vi "Handle Messages.vi"(8 "error in (no error)":errorcluster, 9 "Message Data":variant, 10 "Message":string, 11 "Process In":refnum<class "Debugger.lvclass">) -> (0 "error out":errorcluster, 3 "Process Out":refnum<class "Debugger.lvclass">)   [LabVIEW 2020, in "Debugger.lvclass"]
doc: "This is the core VI handling incomming messages to the process. This VI should be overridden to add functionality to the process or override functionality implemented by a parent. Any message not handled should be sent to the parent method using the default case. \nEach state should be atomic and states should in general avoid enqueueing new messages from within this method, as there might be other messages interleaved in the queue from the outside. For cyclic iteration of an action, using a Helper Loop is recommended."
uses:
  Debugger.lvclass
  C:/Git/astemes-triarc-debugger/source/Process/Debug Process.lvclass
  Debug Data/Debug Data.lvclass
  Debugger.lvclass/Debugger.ctl
  Debug Log/Debug Log.lvclass/Debug Log.ctl
  Process/Debug Process.lvclass/Debug Process.ctl
  Process/Public/Lifecycle/Get Lifecycle State.vi
  <vilib>/Utility/error.llb/Clear Errors.vi
  <vilib>/Utility/error.llb/Error Cluster From Error Code.vi
  Process/Debug Process.lvclass
  Debug Log/Debug Log.lvclass
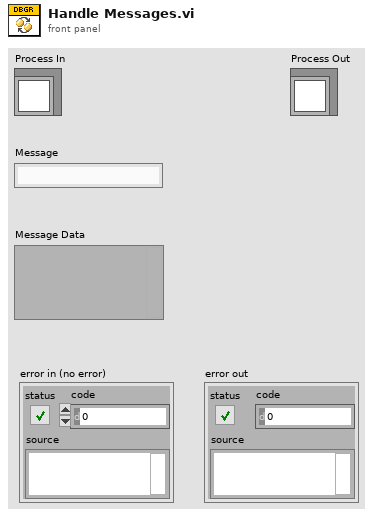
[diagram p1: front panel]
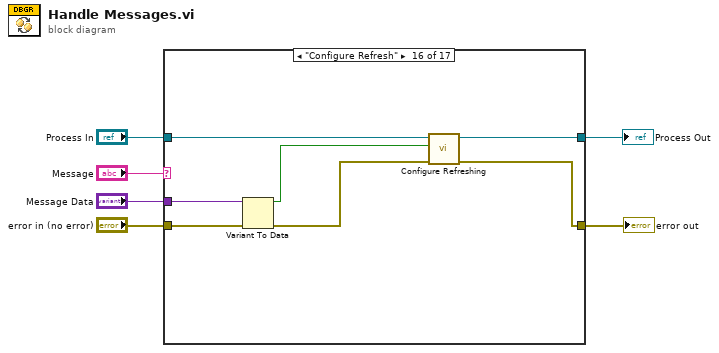
[diagram p0: block diagram]
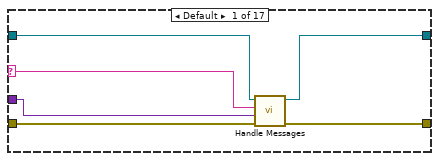
[diagram p2: hidden frame]
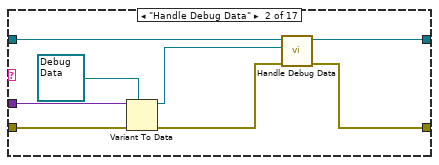
[diagram p3: hidden frame]
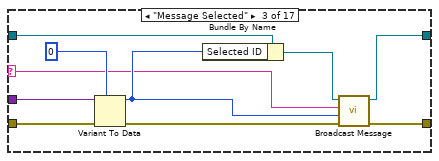
[diagram p4: hidden frame]
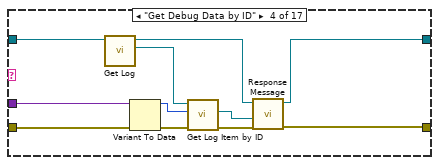
[diagram p5: hidden frame]
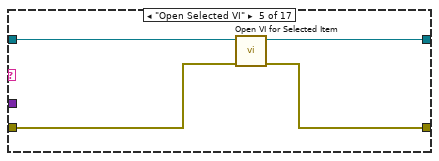
[diagram p6: hidden frame]
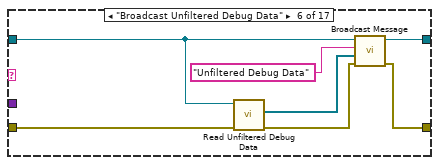
[diagram p7: hidden frame]
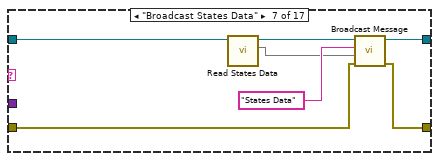
[diagram p8: hidden frame]
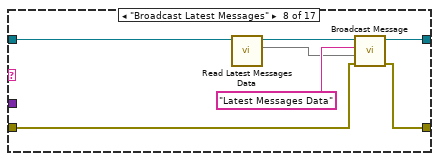
[diagram p9: hidden frame]
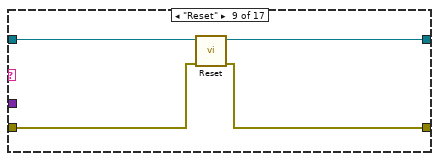
[diagram p10: hidden frame]
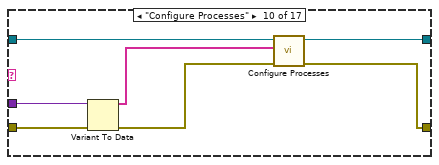
[diagram p11: hidden frame]
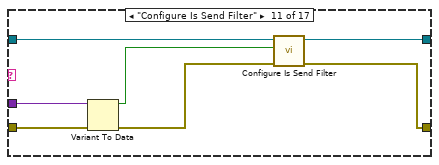
[diagram p12: hidden frame]
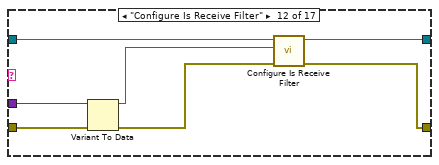
[diagram p13: hidden frame]
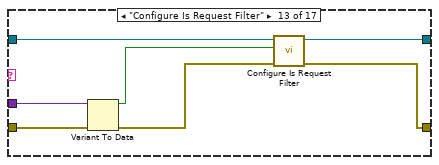
[diagram p14: hidden frame]
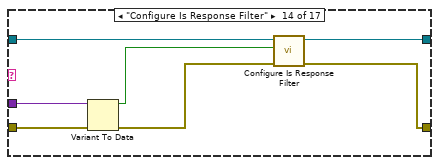
[diagram p15: hidden frame]
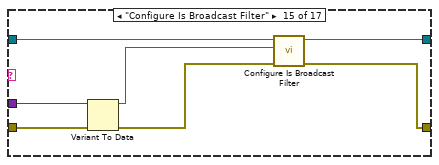
[diagram p16: hidden frame]
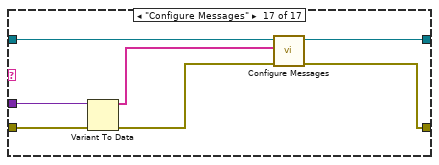
[diagram p17: hidden frame]
diagram:
  n1 = case shown="\"Configure Refresh\"" "Message" {
    selector: "Message" -> [w8 _ w22 _ _ _ _ _ _ _ _ _ _ _ _ _ _]
    tunnel: [w12 w13 w25 w40 w42 w51 w58 w65 w67 w72 w79 w86 w93 w100 w107 w114 w121] -> w6
    tunnel: [w11 w15 w21 w41 w44 w52 w59 w66 w69 w73 w80 w87 w94 w101 w108 w115 w122] -> w5
    tunnel: "error in (no error)" -> [w10 w19 w29 w37 w45 w49 w56 w63 w68 w77 w84 w91 w98 w105 w112 w119 w126]
    tunnel: "Message Data" -> [w9 w20 w30 w38 _ _ _ _ _ w76 w83 w90 w97 w104 w111 w118 w125]
    tunnel: "Process In" -> [w7 w16 w27 w31 w43 w50 w57 w64 w70 w74 w81 w88 w95 w102 w109 w116 w123]
    frame Default {
      n2 = call-parent "Handle Messages.vi"("error in (no error)"=w10, "Message Data"=w9, "Message"=w8, "Process In"=w7) -> ("error out"=w12:errorcluster, "Process Out"=w11:refnum<class "Debugger.lvclass">)  [unwired: 6 in]
    }
    frame "Handle Debug Data" {
      n3 = Variant To Data(error in=w19, type=refnum<class "Debug Data.lvclass"> refnum ("Debug Data.lvclass"), Variant=w20) -> (data=w14:refnum<class "Debug Data.lvclass">, error out=w17:errorcluster)
      n4 = call-dynamic "Handle Debug Data.vi"("error in (no error)"=w17, "Debug Data.lvclass"=w14, "Debug Data Event In"=w16) -> ("error out"=w13:errorcluster, "Debug Data Event Out"=w15:refnum<class "Debugger.lvclass">)  [unwired: 7 in]
    }
    frame "Message Selected" {
      n5 = Variant To Data(error in=w29, type=u32 0 ("Message ID"), Variant=w30) -> (data=w23:u32, error out=w26:errorcluster)
      n6 = Bundle By Name(cluster=w27, "Selected ID"=w23) -> (w24:refnum<class "Debugger.lvclass">)
      n7 = call-dynamic "Broadcast Message.vi"("error in (no error)"=w26, "Message Data"=w23, "Message"=w22, "Process In"=w24) -> ("error out"=w25:errorcluster, "Process Out"=w21:refnum<class "Debugger.lvclass">)  [unwired: 6 in]
    }
    frame "Get Debug Data by ID" {
      n8 = call "Get Log.vi"("Debugger in"=w31) -> ("Log"=w39:refnum<class "Debug Log.lvclass">, "Debugger out"=w32:refnum<class "Debugger.lvclass">)  [unwired: 8 in, 1 out]
      n9 = Variant To Data(error in=w37, Variant=w38) -> (data=w36:u32, error out=w35:errorcluster)  [unwired: 1 in]
      n10 = call "Get Log Item by ID.vi"("error in (no error)"=w35, "ID"=w36, "Debug Log In"=w39) -> ("error out"=w33:errorcluster, "Data Log"=w34:refnum<class "Debug Data.lvclass">)  [unwired: 6 in, 1 out]
      n11 = call "Response Message.vi"("error in (no error)"=w33, "Response Message Data"=w34, "Process In"=w32) -> ("error out"=w40:errorcluster, "Process Out"=w41:refnum<class "Debugger.lvclass">)  [unwired: 7 in]
    }
    frame "Open Selected VI" {
      n12 = call "Open VI for Selected Item.vi"("error in (no error)"=w45, "Debugger In"=w43) -> ("error out"=w42:errorcluster, "Debugger Out"=w44:refnum<class "Debugger.lvclass">)  [unwired: 8 in]
    }
    frame "Broadcast Unfiltered Debug Data" {
      n13 = call "Read Unfiltered Debug Data.vi"("error in (no error)"=w49, "Debugger In"=w50) -> ("error out"=w47:errorcluster, "Data Log"=w46:refnum<class "Debug Data.lvclass">[])  [unwired: 7 in, 1 out]
      n14 = call-dynamic "Broadcast Message.vi"("error in (no error)"=w47, "Message Data"=w46, "Message"="Unfiltered Debug Data", "Process In"=w50) -> ("error out"=w51:errorcluster, "Process Out"=w52:refnum<class "Debugger.lvclass">)  [unwired: 6 in]
    }
    frame "Broadcast States Data" {
      n15 = call "Read States Data.vi"("Debugger in"=w57) -> ("State Map"=w54:map{string, string}, "Debugger in 2"=w53:refnum<class "Debugger.lvclass">)  [unwired: 8 in, 1 out]
      n16 = call-dynamic "Broadcast Message.vi"("error in (no error)"=w56, "Message Data"=w54, "Message"="States Data", "Process In"=w53) -> ("error out"=w58:errorcluster, "Process Out"=w59:refnum<class "Debugger.lvclass">)  [unwired: 6 in]
    }
    frame "Broadcast Latest Messages" {
      n17 = call "Read Latest Messages Data.vi"("Debugger In"=w64) -> ("Latest Messages"=w60:map{string, refnum<class "Debug Data.lvclass">}, "Debugger Out"=w61:refnum<class "Debugger.lvclass">)  [unwired: 8 in, 1 out]
      n18 = call-dynamic "Broadcast Message.vi"("error in (no error)"=w63, "Message Data"=w60, "Message"="Latest Messages Data", "Process In"=w61) -> ("error out"=w65:errorcluster, "Process Out"=w66:refnum<class "Debugger.lvclass">)  [unwired: 6 in]
    }
    frame "Reset" {
      n19 = call "Reset.vi"("error in (no error)"=w68, "Debugger in"=w70) -> ("error out"=w67:errorcluster, "Debugger out"=w69:refnum<class "Debugger.lvclass">)  [unwired: 8 in]
    }
    frame "Configure Processes" {
      n20 = Variant To Data(error in=w77, Variant=w76) -> (data=w75:string[], error out=w71:errorcluster)  [unwired: 1 in]
      n21 = call "Configure Processes.vi"("error in (no error)"=w71, "Processes"=w75, "Debugger In"=w74) -> ("error out"=w72:errorcluster, "Debugger Out"=w73:refnum<class "Debugger.lvclass">)  [unwired: 7 in]
    }
    frame "Configure Is Send Filter" {
      n22 = Variant To Data(error in=w84, Variant=w83) -> (data=w82:bool, error out=w78:errorcluster)  [unwired: 1 in]
      n23 = call "Configure Is Send Filter.vi"("error in (no error)"=w78, "Show Send?"=w82, "Debugger In"=w81) -> ("error out"=w79:errorcluster, "Debugger Out"=w80:refnum<class "Debugger.lvclass">)  [unwired: 7 in]
    }
    frame "Configure Is Receive Filter" {
      n24 = Variant To Data(error in=w91, Variant=w90) -> (data=w89:bool, error out=w85:errorcluster)  [unwired: 1 in]
      n25 = call "Configure Is Receive Filter.vi"("error in (no error)"=w85, "Show Receive?"=w89, "Debugger In"=w88) -> ("error out"=w86:errorcluster, "Debugger Out"=w87:refnum<class "Debugger.lvclass">)  [unwired: 7 in]
    }
    frame "Configure Is Request Filter" {
      n26 = Variant To Data(error in=w98, Variant=w97) -> (data=w96:bool, error out=w92:errorcluster)  [unwired: 1 in]
      n27 = call "Configure Is Request Filter.vi"("error in (no error)"=w92, "Show Request?"=w96, "Debugger In"=w95) -> ("error out"=w93:errorcluster, "Debugger Out"=w94:refnum<class "Debugger.lvclass">)  [unwired: 7 in]
    }
    frame "Configure Is Response Filter" {
      n28 = Variant To Data(error in=w105, Variant=w104) -> (data=w103:bool, error out=w99:errorcluster)  [unwired: 1 in]
      n29 = call "Configure Is Response Filter.vi"("error in (no error)"=w99, "Show Response?"=w103, "Debugger In"=w102) -> ("error out"=w100:errorcluster, "Debugger Out"=w101:refnum<class "Debugger.lvclass">)  [unwired: 7 in]
    }
    frame "Configure Is Broadcast Filter" {
      n30 = Variant To Data(error in=w112, Variant=w111) -> (data=w110:bool, error out=w106:errorcluster)  [unwired: 1 in]
      n31 = call "Configure Is Broadcast Filter.vi"("error in (no error)"=w106, "Show Broadcast?"=w110, "Debugger In"=w109) -> ("error out"=w107:errorcluster, "Debugger Out"=w108:refnum<class "Debugger.lvclass">)  [unwired: 7 in]
    }
    frame "Configure Refresh" {
      n32 = Variant To Data(error in=w119, Variant=w118) -> (data=w117:bool, error out=w113:errorcluster)  [unwired: 1 in]
      n33 = call "Configure Refreshing.vi"("error in (no error)"=w113, "Refresh?"=w117, "Debugger In"=w116) -> ("error out"=w114:errorcluster, "Debugger Out"=w115:refnum<class "Debugger.lvclass">)  [unwired: 7 in]
    }
    frame "Configure Messages" {
      n34 = Variant To Data(error in=w126, Variant=w125) -> (data=w124:string[], error out=w120:errorcluster)  [unwired: 1 in]
      n35 = call "Configure Messages.vi"("error in (no error)"=w120, "Messages"=w124, "Debugger In"=w123) -> ("error out"=w121:errorcluster, "Debugger Out"=w122:refnum<class "Debugger.lvclass">)  [unwired: 7 in]
    }
  }
  "error out" <- w6
  "Process Out" <- w5
